vi "RUSHControls.vi"() -> (1 "Harvester":dbl, 2 "Conveyor":dbl)   [LabVIEW 2011]
uses:
  GLOBALDriver.vi
  GLOBALBridge.vi
  GLOBALHarvester.vi
  GLOBALShooter.vi
panel:
  out "Button 5":bool
  out "Button 7":bool
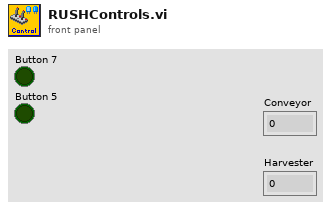
[diagram p1: front panel]
types:
  T1 = cluster{"Driver Station Digital Input (1-8)[0]":bool, "Driver Station Digital Input (1-8)[1]":bool, "Driver Station Digital Input (1-8)[2]":bool, "Driver Station Digital Input (1-8)[3]":bool, "Driver Station Digital Input (1-8)[4]":bool, "Driver Station Digital Input (1-8)[5]":bool, "Driver Station Digital Input (1-8)[6]":bool, "Driver Station Digital Input (1-8)[7]":bool, "Driver Station Digital Input (1-8)[8]":bool}
  T2 = typedef "WPI_JoystickDevRef.ctl" = cluster{"Device":T3}
  T3 = typedef "WPI_JoystickDeviceEnum.ctl" = enum16{"USB 1", "USB 2", "USB 3", "USB 4", "Kinect 1", "Kinect 2"}
  T4 = typedef "WPI_JoystickButtonState.ctl" = cluster{"Button 1":bool, "Button 2":bool, "Button 3":bool, "Button 4":bool, "Button 5":bool, "Button 6":bool, "Button 7":bool, "Button 8":bool, "Button 9":bool, "Button 10":bool, "Button 11":bool, "Button 12":bool}
  T5 = cluster{"axis 1 (x)":dbl, "axis 2 (y)":dbl, "axis 3 (throttle)":dbl, "axis 4":dbl, "axis 5":dbl, "axis 6":dbl}
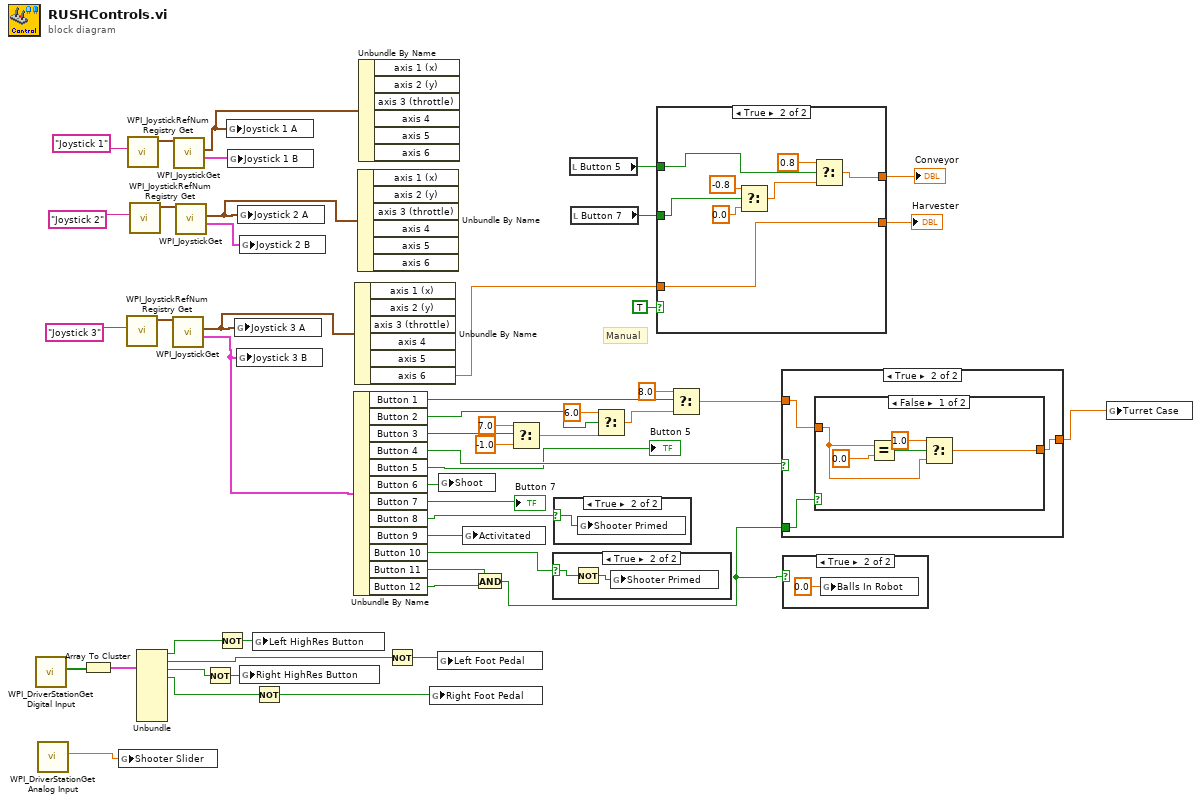
[diagram p0: block diagram]
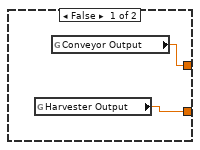
[diagram p2: hidden frame]
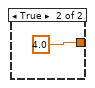
[diagram p5: hidden frame]
diagram:
  # "Manual"
  n1 = call <vilib>:"WPI_DriverStationGet Digital Input.vi"() -> ("Driver Station Digital Input (1-8)"=w45:bool[])  [unwired: 11 in]
  n2 = call <vilib>:"WPI_DriverStationGet Analog Input.vi"() -> ("Analog 2 (V)"=w43:dbl)  [unwired: 8 in, 3 out]
  n3 = Array To Cluster(array=w45) -> (cluster=w44:T1)
  n4 = global write "GLOBALDriver.vi" "Shooter Slider"(w43) -> ()
  n5 = call <vilib>:"WPI_JoystickRefNum Registry Get.vi"("refnum name"="Joystick 3" ("Joystick 2")) -> ("JoystickDevRef"=w38:T2)  [unwired: 9 in, 1 out]
  n6 = call <vilib>:"WPI_JoystickRefNum Registry Get.vi"("refnum name"="Joystick 1" ("Joystick 1")) -> ("JoystickDevRef"=w50:T2)  [unwired: 9 in, 1 out]
  n7 = call <vilib>:"WPI_JoystickRefNum Registry Get.vi"("refnum name"="Joystick 2" ("Joystick 2")) -> ("JoystickDevRef"=w46:T2)  [unwired: 9 in, 1 out]
  n8 = Unbundle(w44) -> ("Driver Station Digital Input (1-8)[0]"=w22:bool, "Driver Station Digital Input (1-8)[1]"=w3:bool, "Driver Station Digital Input (1-8)[2]"=w24:bool, "Driver Station Digital Input (1-8)[3]"=w2:bool)  [unwired: 5 out]
  n9 = call <vilib>:"WPI_JoystickGet.vi"("JoystickDevRef"=w38) -> ("Buttons"=w36:T4, "Axes"=w39:T5)  [unwired: 4 in, 1 out]
  n10 = call <vilib>:"WPI_JoystickGet.vi"("JoystickDevRef"=w50) -> ("Buttons"=w42:T4, "Axes"=w41:T5)  [unwired: 4 in, 1 out]
  n11 = call <vilib>:"WPI_JoystickGet.vi"("JoystickDevRef"=w46) -> ("Buttons"=w48:T4, "Axes"=w40:T5)  [unwired: 4 in, 1 out]
  n12 = Not(x=w24) -> (.not. x?=w25:bool)
  n13 = Not(x=w22) -> (.not. x?=w23:bool)
  n14 = global write "GLOBALDriver.vi" "Joystick 1 A"(w41) -> ()
  n15 = global write "GLOBALDriver.vi" "Joystick 1 B"(w42) -> ()
  n16 = global write "GLOBALDriver.vi" "Joystick 3 A"(w39) -> ()
  n17 = global write "GLOBALDriver.vi" "Joystick 3 B"(w36) -> ()
  n18 = global write "GLOBALDriver.vi" "Joystick 2 A"(w40) -> ()
  n19 = global write "GLOBALDriver.vi" "Joystick 2 B"(w48) -> ()
  n20 = global write "GLOBALDriver.vi" "Right HighRes Button"(w25) -> ()
  n21 = global write "GLOBALDriver.vi" "Left HighRes Button"(w23) -> ()
  n22 = Not(x=w2) -> (.not. x?=w1:bool)
  n23 = Unbundle By Name(w36) -> ("Button 1"=w35:bool, "Button 2"=w34:bool, "Button 3"=w33:bool, "Button 4"=w19:bool, "Button 5"=→"Button 5":bool, "Button 6"=w13:bool, "Button 7"=→"Button 7":bool, "Button 8"=w21:bool, "Button 9"=w26:bool, "Button 10"=w20:bool, "Button 11"=w18:bool, "Button 12"=w17:bool)
  n24 = Unbundle By Name(w39) -> ("axis 6"=w5:dbl)  [unwired: 5 out]
  n25 = Unbundle By Name(w40) -> ()  [unwired: 6 out]
  n26 = Unbundle By Name(w41) -> ()  [unwired: 6 out]
  n27 = Not(x=w3) -> (.not. x?=w4:bool)
  n28 = global write "GLOBALDriver.vi" "Right Foot Pedal"(w1) -> ()
  n29 = global write "GLOBALDriver.vi" "Left Foot Pedal"(w4) -> ()
  n30 = global write "GLOBALHarvester.vi" "Shoot"(w13) -> ()
  n31 = global write "GLOBALBridge.vi" "Activitated"(w26) -> ()
  n32 = And(x=w18, y=w17) -> (x .and. y?=w14:bool)
  n33 = Select(t=7.0, s=w33, f=-1.0) -> (s? t:f=w31:dbl)
  n34 = case shown="True" w20 {
    selector: w20 -> [_ w52]
    frame False {
    }
    frame True {
      n35 = Not(x=w52) -> (.not. x?=w51:bool)
      n36 = global write "GLOBALShooter.vi" "Shooter Primed"(w51) -> ()
    }
  }
  n37 = case shown="True" w21 {
    selector: w21 -> [_ w53]
    frame False {
    }
    frame True {
      n38 = global write "GLOBALShooter.vi" "Shooter Primed"(w53) -> ()
    }
  }
  n39 = local read "Button 5"() -> (w9:bool)
  n40 = local read "Button 7"() -> (w8:bool)
  n41 = Select(t=6.0, s=w34, f=w31) -> (s? t:f=w32:dbl)
  n42 = case shown="True" TRUE {
    tunnel: w9 -> [_ w59]
    tunnel: w8 -> [_ w58]
    tunnel: [w55 w57] -> w7
    tunnel: [w54 w56] -> w6
    tunnel: w5 -> [_ w56]
    frame False {
      n43 = global read "GLOBALHarvester.vi" "Harvester Output"() -> (w54:dbl)
      n44 = global read "GLOBALHarvester.vi" "Conveyor Output"() -> (w55:dbl)
    }
    frame True {
      n45 = Select(t=-0.8, s=w58, f=0.0) -> (s? t:f=w60:dbl)
      n46 = Select(t=0.8, s=w59, f=w60) -> (s? t:f=w57:dbl)
    }
  }
  "Conveyor" <- w7
  "Harvester" <- w6
  n47 = Select(t=8.0, s=w35, f=w32) -> (s? t:f=w16:dbl)
  n48 = case shown="True" w19 {
    tunnel: w14 -> [_ w67]
    tunnel: w16 -> [w64 w66]
    tunnel: [w64 w65] -> w15
    frame False {
    }
    frame True {
      n49 = case shown="False" w67 {
        tunnel: w66 -> [w70 _]
        tunnel: [w68 4.0 ("f")] -> w65
        frame False {
          n50 = Equal?(x=w70, y=0.0) -> (x = y?=w71:bool)
          n51 = Select(t=1.0, s=w71, f=w70) -> (s? t:f=w68:dbl)
        }
        frame True {
        }
      }
    }
  }
  n52 = case shown="True" w14 {
    frame False {
    }
    frame True {
      n53 = global write "GLOBALHarvester.vi" "Balls In Robot"(0.0 ("Balls In Robot")) -> ()
    }
  }
  n54 = global write "GLOBALShooter.vi" "Turret Case"(w15) -> ()
